vi "Test Constructor.vi"(8 "error in":errorcluster, 11 "data":T1) -> (0 "error out":errorcluster, 3 "session reservation out":refnum<class "Session Reservation.lvclass">)   [LabVIEW 2020, in "MeasurementLink Session Management.lvlib" / "Session Reservation.lvclass"]
uses:
  Session Reservation.lvclass
  Data.ctl
  Connection Map/Connection Map.lvclass
  IReservationObserver/IReservationObserver.lvclass
  Session and Driver Info.ctl
  MeasurementLink Instrument/ISession Factory/ISession Factory.lvclass
  MeasurementLink Session Management Client/RPC Messages/ni_measurementlink_sessionmanagement_v1_SessionInformation.ctl
  MeasurementLink Session Management Client/RPC Messages/nidevice_grpc_Session.ctl
  MeasurementLink Session Management Client/RPC Messages/ni_measurementlink_sessionmanagement_v1_ChannelMapping.ctl
  MeasurementLink Instrument/ISession Factory/Initialize and Close Session Behavior.ctl
  MeasurementLink Session Management Client/RPC Messages/ni_measurementlink_PinMapContext.ctl
  Session Reservation.lvclass/Session Reservation.ctl
  MeasurementLink Session Management Client/MeasurementLink Session Management Client.lvlib
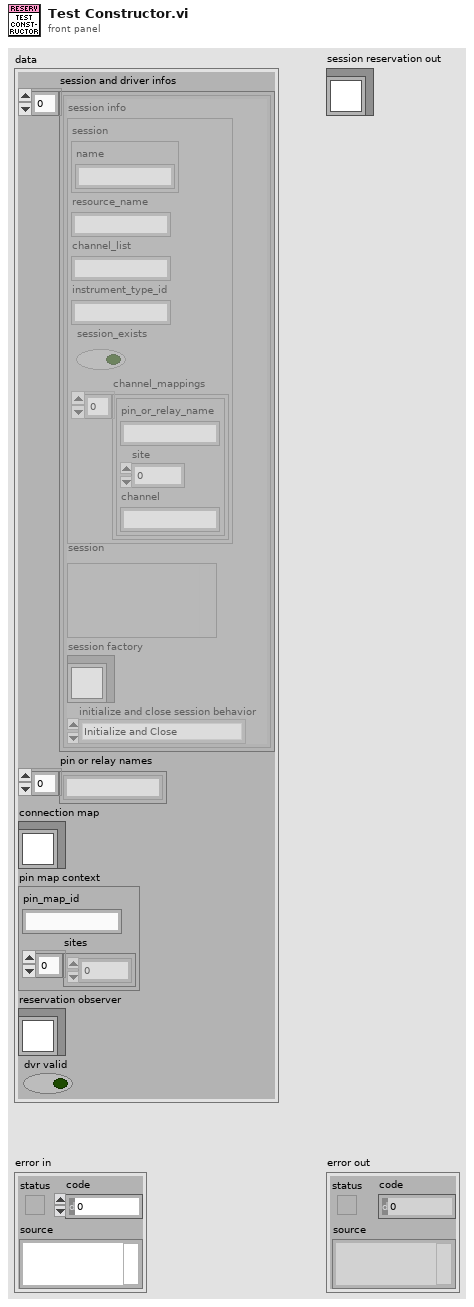
[diagram p1: front panel]
types:
  T1 = typedef "MeasurementLink Session Management.lvlib/Session Reservation.lvclass/Data.ctl" = cluster{"session and driver infos":T2[], "pin or relay names":string[], "connection map":refnum<class "Connection Map.lvclass">, "pin map context":T7, "reservation observer":refnum<class "IReservationObserver.lvclass">, "dvr valid":bool}
  T2 = typedef "MeasurementLink Session Management.lvlib/Session Reservation.lvclass/Session and Driver Info.ctl" = cluster{"session info":T3, "session":variant, "session factory":refnum<class "ISession Factory.lvclass">, "initialize and close session behavior":T6}
  T3 = typedef "MeasurementLink Session Management Client.lvlib/ni_measurementlink_sessionmanagement_v1_SessionInformation.ctl" = cluster{"session":T4, "resource_name":string, "channel_list":string, "instrument_type_id":string, "session_exists":bool, "channel_mappings":T5[]}
  T4 = typedef "MeasurementLink Session Management Client.lvlib/nidevice_grpc_Session.ctl" = cluster{"name":string}
  T5 = typedef "MeasurementLink Session Management Client.lvlib/ni_measurementlink_sessionmanagement_v1_ChannelMapping.ctl" = cluster{"pin_or_relay_name":string, "site":i32, "channel":string}
  T6 = typedef "MeasurementLink Instrument.lvlib/ISession Factory.lvclass/Initialize and Close Session Behavior.ctl" = enum16{"Initialize and Close", "Attach and Detach", "Initialize and Detach", "Attach and Close"}
  T7 = typedef "MeasurementLink Session Management Client.lvlib/ni_measurementlink_PinMapContext.ctl" = cluster{"pin_map_id":string, "sites":i32[]}
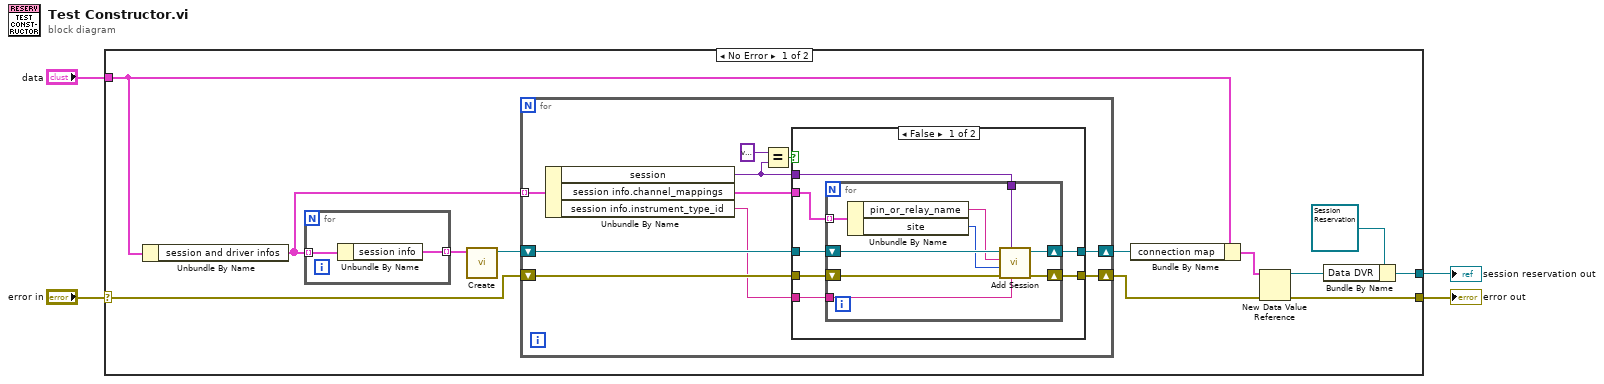
[diagram p0: block diagram]
diagram:
  n1 = case shown="No Error" "error in" {
    selector: "error in" -> [w7 w47]
    tunnel: [w14 w47] -> w3
    tunnel: "data" -> [w11 _]
    tunnel: [w13 _] -> w1
    frame No Error {
      n2 = Unbundle By Name(w11) -> ("session and driver infos"=w9:T2[])
      n3 = for {
        tunnel: w9 -> [w46] mode=indexing
        tunnel: [w45] -> w12 mode=indexing
        n4 = Unbundle By Name(w46) -> ("session info"=w45:T3)
      }
      n5 = call "Create.vi"("session info"=w12) -> ("connection map"=w8:refnum<class "Connection Map.lvclass">)  [unwired: 10 in]
      n6 = for {
        tunnel: w9 -> [w26] mode=indexing
        shift-right: [w22] -> w5
        shift-left: w8 -> [w24]
        shift-right: [w20] -> w6
        shift-left: w7 -> [w21]
        n7 = Unbundle By Name(w26) -> ("session"=w19:variant, "session info.channel_mappings"=w18:T5[], "session info.instrument_type_id"=w17:string)
        n8 = Equal?(x=variant ("session"), y=w19) -> (x = y?=w23:bool)
        n9 = case shown="False" w23 {
          tunnel: w24 -> [w33 w44]
          tunnel: [w32 w44] -> w22
          tunnel: w21 -> [w31 w43]
          tunnel: [w30 w43] -> w20
          tunnel: w19 -> [w29 _]
          tunnel: w18 -> [w27 _]
          tunnel: w17 -> [w28 _]
          frame False {
            n10 = for {
              tunnel: w29 -> [w38]
              tunnel: w28 -> [w37]
              shift-right: [w41] -> w32
              shift-left: w33 -> [w42]
              shift-right: [w39] -> w30
              shift-left: w31 -> [w40]
              tunnel: w27 -> [w36] mode=indexing
              n11 = Unbundle By Name(w36) -> ("pin_or_relay_name"=w35:string, "site"=w34:i32)
              n12 = call "Add Session.vi"("instrument type id"=w37, "session to add"=w38, "error in"=w40, "site"=w34, "pin or relay name"=w35, "connection map in"=w42) -> ("error out"=w39:errorcluster, "connection map out"=w41:refnum<class "Connection Map.lvclass">)  [unwired: 4 in]
            }
          }
          frame True {
          }
        }
      }
      n13 = Bundle By Name(cluster=w11, "connection map"=w5) -> (w10:T1)
      n14 = New Data Value Reference(data value=w10, error in=w6) -> (data value reference=w15:refnum<data-value>, error out=w14:errorcluster)
      n15 = Bundle By Name(cluster=refnum<class "Session Reservation.lvclass"> refnum ("MeasurementLink Session Management.lvlib:Session Reservation.lvclass"), "Data DVR"=w15) -> (w13:refnum<class "Session Reservation.lvclass">)
    }
    frame Error {
    }
  }
  "error out" <- w3
  "session reservation out" <- w1
